vi "Load Network from File.vi"(5 "File Path (dialog)":path, 11 "Error In":errorcluster) -> (4 "Neural Network Out":refnum<class "Neural Network.lvclass">, 6 "Used Path":path, 10 "Cancelled":bool, 15 "Error Out":errorcluster)   [LabVIEW 2015, in "Neural Network.lvclass"]
doc: "Load neural network from a user editable INI file."
uses:
  Neural Network.lvclass
  <vilib>/Utility/config.llb/NI_LVConfig.lvlib
  Types/2D Array.ctl
  <vilib>/Utility/config.llb/Read Key (U32).vi
  <vilib>/Utility/config.llb/Read Key (String).vi
  <vilib>/Utility/config.llb/Read Key (Boolean).vi
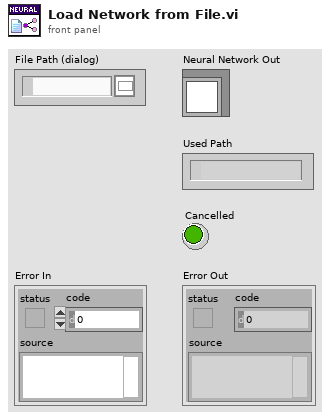
[diagram p1: front panel]
types:
  T1 = typedef "Neural Network.lvclass/2D Array.ctl" = cluster{"2D Array":sgl[][]}
  T2 = typedef "NI_LVConfig.lvlib/Config Data RefNum.ctl" = refnum<k1>
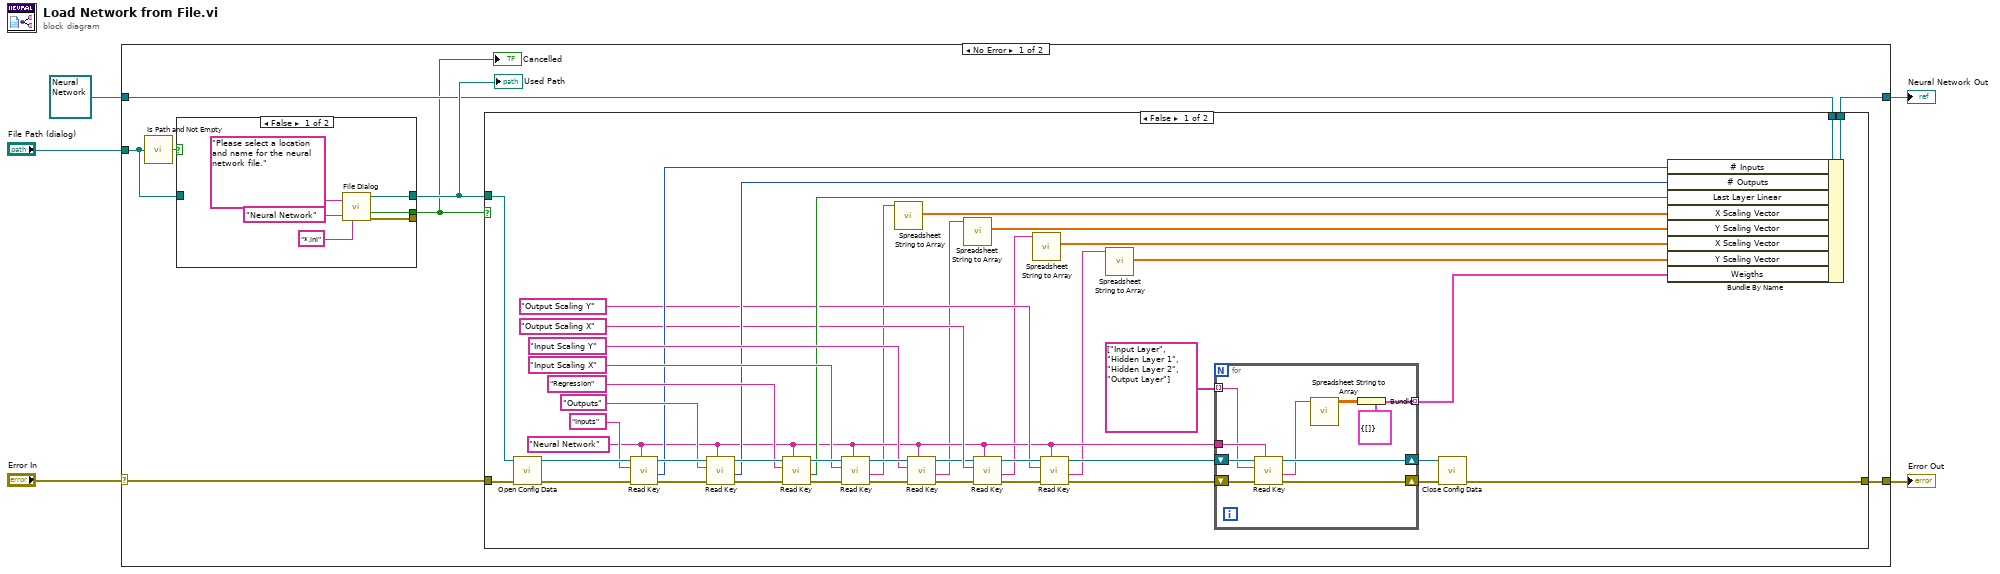
[diagram p0: block diagram]
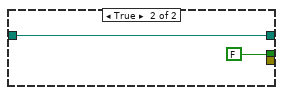
[diagram p3: hidden frame]
diagram:
  n1 = case shown="No Error" "Error In" {
    selector: "Error In" -> [w11 w79]
    tunnel: [w9 w79] -> w4
    tunnel: [w6 w78] -> w2
    tunnel: refnum<class "Neural Network.lvclass"> refnum ("Neural Network In") -> [w10 w78]
    tunnel: "File Path (dialog)" -> [w8 _]
    frame No Error {
      n2 = call <vilib>:"Is Path and Not Empty.vi"("path"=w8) -> ("Is Path and Not Empty?"=w13:bool)  [unwired: 4 in]
      n3 = case shown="False" w13 {
        tunnel: [w72 w77] -> w12
        tunnel: w8 -> [_ w77]
        tunnel: [w71 FALSE ("cancelled")] -> w7
        tunnel: [w70 _] -> _
        frame False {
          n4 = call "File Dialog"("prompt"="Please select a location and name for the neural network file.", "pattern (all files)"="*.ini", "pattern label"="Neural Network") -> ("selected path"=w72:path, "cancelled"=w71:bool, "error out"=w70:errorcluster)  [unwired: 9 in, 1 out]
        }
        frame True {
        }
      }
      "Cancelled" <- w7
      "Used Path" <- w12
      n5 = case shown="False" w7 {
        tunnel: w12 -> [w39 _]
        tunnel: w11 -> [w38 w69]
        tunnel: w10 -> [w37 w68]
        tunnel: [w32 w69] -> w9
        tunnel: [w36 w68] -> w6
        frame False {
          w22 = "Neural Network" ("section")
          n6 = call <vilib>:"Open Config Data.vi"("error in (no error)"=w38, "configuration file path"=w39) -> ("error out"=w56:errorcluster, "refnum"=w57:T2)  [unwired: 7 in, 1 out]
          n7 = call-poly <vilib>:"Read Key.vi"("section"=w22, "error in (no error)"=w56, "key"="Inputs", "refnum"=w57) -> ("error out"=w54:errorcluster, "value"=w34:u32, "refnum out"=w55:T2)  [unwired: 4 in, 1 out]
          n8 = call-poly <vilib>:"Read Key.vi"("section"=w22, "error in (no error)"=w54, "key"="Outputs", "refnum"=w55) -> ("error out"=w50:errorcluster, "value"=w33:u32, "refnum out"=w51:T2)  [unwired: 4 in, 1 out]
          n9 = call-poly <vilib>:"Read Key.vi"("section"=w22, "error in (no error)"=w50, "key"="Regression", "refnum"=w51) -> ("error out"=w49:errorcluster, "value"=w31:bool, "refnum out"=w46:T2)  [unwired: 4 in, 1 out]
          n10 = call-poly <vilib>:"Read Key.vi"("section"=w22, "error in (no error)"=w49, "key"="Input Scaling X", "refnum"=w46) -> ("error out"=w47:errorcluster, "value"=w21:string, "refnum out"=w44:T2)  [unwired: 4 in, 1 out]
          n11 = call "Spreadsheet String to Array.vi"("Spreadsheet String"=w21) -> ("1D Array"=w20:dbl[])  [unwired: 9 in, 1 out]
          n12 = call-poly <vilib>:"Read Key.vi"("section"=w22, "error in (no error)"=w47, "key"="Input Scaling Y", "refnum"=w44) -> ("error out"=w28:errorcluster, "value"=w19:string, "refnum out"=w29:T2)  [unwired: 4 in, 1 out]
          n13 = call "Spreadsheet String to Array.vi"("Spreadsheet String"=w19) -> ("1D Array"=w18:dbl[])  [unwired: 9 in, 1 out]
          n14 = call-poly <vilib>:"Read Key.vi"("section"=w22, "error in (no error)"=w28, "key"="Output Scaling X", "refnum"=w29) -> ("error out"=w27:errorcluster, "value"=w17:string, "refnum out"=w26:T2)  [unwired: 4 in, 1 out]
          n15 = call "Spreadsheet String to Array.vi"("Spreadsheet String"=w17) -> ("1D Array"=w16:dbl[])  [unwired: 9 in, 1 out]
          n16 = call-poly <vilib>:"Read Key.vi"("section"=w22, "error in (no error)"=w27, "key"="Output Scaling Y", "refnum"=w26) -> ("error out"=w23:errorcluster, "value"=w15:string, "refnum out"=w24:T2)  [unwired: 4 in, 1 out]
          n17 = call "Spreadsheet String to Array.vi"("Spreadsheet String"=w15) -> ("1D Array"=w14:dbl[])  [unwired: 9 in, 1 out]
          n18 = for {
            shift-right: [w66] -> w42
            shift-left: w23 -> [w67]
            shift-right: [w64] -> w41
            shift-left: w24 -> [w65]
            tunnel: w22 -> [w63]
            tunnel: string[] ["Input Layer", "Hidden Layer 1", "Hidden Layer 2", "Output Layer"] -> [w62] mode=indexing
            tunnel: [w60] -> w35 mode=indexing
            n19 = call-poly <vilib>:"Read Key.vi"("section"=w63, "error in (no error)"=w67, "key"=w62, "refnum"=w65) -> ("error out"=w66:errorcluster, "value"=w59:string, "refnum out"=w64:T2)  [unwired: 4 in, 1 out]
            n20 = call "Spreadsheet String to Array.vi"("Spreadsheet String"=w59) -> ("2D Array"=w58:dbl[][])  [unwired: 9 in, 1 out]
            n21 = Bundle(cluster=T1 {"2D Array"=[]}, "2D Array"=w58) -> (w60:T1)
          }
          n22 = call <vilib>:"Close Config Data.vi"("error in (no error)"=w42, "refnum"=w41) -> ("error out"=w32:errorcluster)  [unwired: 8 in, 1 out]
          n23 = Bundle By Name(cluster=w37, "# Inputs"=w34, "# Outputs"=w33, "Last Layer Linear"=w31, "X Scaling Vector"=w20, "Y Scaling Vector"=w18, "X Scaling Vector"=w16, "Y Scaling Vector"=w14, "Weigths"=w35) -> (w36:refnum<class "Neural Network.lvclass">)
        }
        frame True {
        }
      }
    }
    frame Error {
    }
  }
  "Error Out" <- w4
  "Neural Network Out" <- w2
